vi "AH2700_Queue_Commands.vi"(1 "AH2700-Control":T1, 3 "AH2700 Queue":refnum<queue> caption="5T Queue") -> (0 "New Status":T1)   [LabVIEW 2019]
uses:
  AH2700/AH2700-Control.ctl
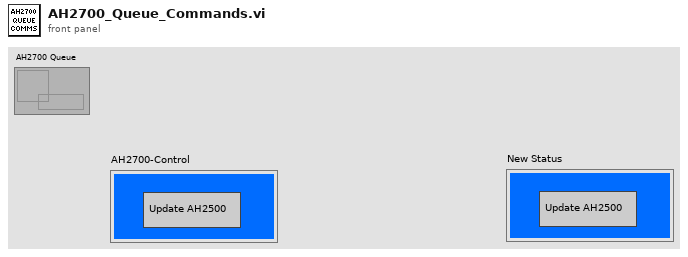
[diagram p1: front panel]
types:
  T1 = typedef "AH2700-Control.ctl" = cluster{"Update AH2500":bool}
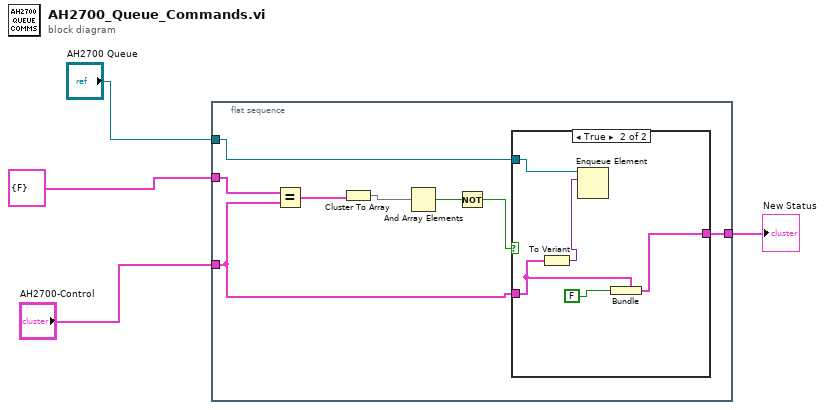
[diagram p0: block diagram]
diagram:
  n1 = flat-sequence {
    tunnel: "AH2700-Control" -> [w6]
    tunnel: T1 {"Update AH2500"=FALSE} ("AH2700-Control") -> [w12]
    tunnel: "AH2700 Queue" -> [w8]
    tunnel: [w5] -> w1
    frame #0 {
      n2 = Equal?(x=w12, y=w6) -> (x = y?=w11:T1)
      n3 = Cluster To Array(cluster=w11) -> (array=w10:bool[])
      n4 = And Array Elements(Boolean array=w10) -> (logical AND=w9:bool)
      n5 = Not(x=w9) -> (.not. x?=w7:bool)
      n6 = case shown="True" w7 {
        tunnel: w8 -> [_ w18]
        tunnel: w6 -> [w13 w16]
        tunnel: [w13 w14] -> w5
        frame False {
        }
        frame True {
          n7 = To Variant(anything=w16) -> (Variant=w17:variant)
          n8 = Enqueue Element(queue=w18, element=w17) -> ()  [unwired: 2 in, 3 out]
          n9 = Bundle(cluster=w16, "Update AH2500"=FALSE) -> (w14:T1)
        }
      }
    }
  }
  "New Status" <- w1
